vi "jl-script examples base path.vi"(8 "error in (no error)":errorcluster, 10 "calling example VI path":path=path "") -> (0 "error out":errorcluster, 1 "jl-script-examples base path":path)   [LabVIEW 2018, in "LV2Julia_core.lvlib"]
doc: "If abs path is connected, this VI only checks if this file exists and puts the path through.\nFor a relative path, the abs path is constructed using the base path. \nIf base path not connected, the containing folder is assumed to be the \"jl-scripts\" folder in this LabVIEW library."
uses:
  LV2Julia_core.lvlib
  <vilib>/Utility/error.llb/Error Cluster From Error Code.vi
  <vilib>/ErrorRing/Error Ring.xnode
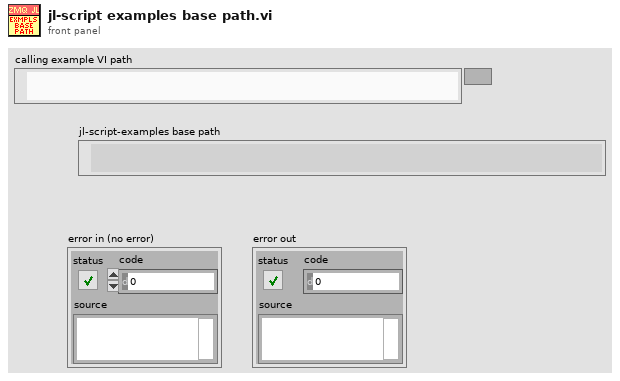
[diagram p1: front panel]
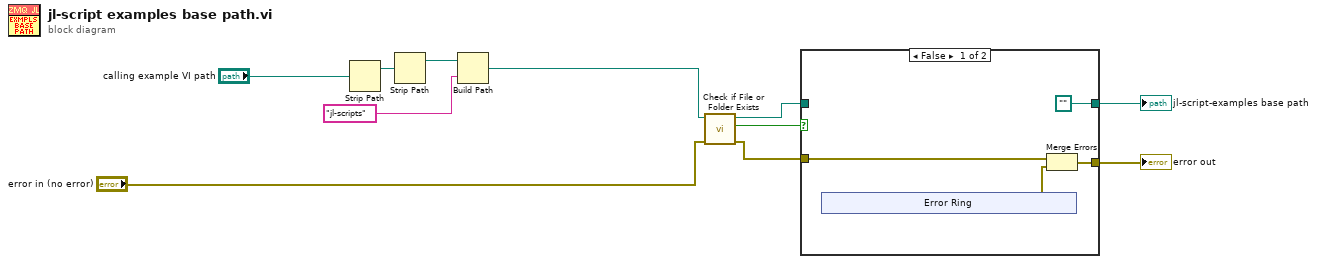
[diagram p0: block diagram]
diagram:
  n1 = Strip Path(path="calling example VI path") -> (stripped path=w4:path)  [unwired: 1 out]
  n2 = Strip Path(path=w4) -> (stripped path=w3:path)  [unwired: 1 out]
  n3 = Build Path(base path=w3, name or relative path="jl-scripts") -> (appended path=w5:path)
  n4 = call <vilib>:"Check if File or Folder Exists.vi"("error in (no error)"="error in (no error)", "path"=w5) -> ("error out"=w9:errorcluster, "file or folder exists?"=w11:bool, "dup path"=w10:path)  [unwired: 7 in]
  n5 = case shown="False" w11 {
    tunnel: w10 -> [_ w22]
    tunnel: [w14 w21] -> w6
    tunnel: w9 -> [w13 w21]
    tunnel: [path "" w22] -> w7
    frame False {
      n6 = xnode "Error Ring"() -> ("error out"=w15:errorcluster)
      n7 = Merge Errors(w13, w15) -> (w14:errorcluster)
    }
    frame True {
      # "script file exists"
    }
  }
  "jl-script-examples base path" <- w7
  "error out" <- w6
